vi "Test_UserEvent.vi"() -> (2 "Tests":cluster{"Test":string, "Passed":bool}[](array[cluster]), 3 "All Passed":bool)   [LabVIEW 2021]
uses:
  e99ad325-cf06-43e8-8912-3f55b24ea7fa.vi
  a4f08420-5a93-4bb2-8b8a-0d8211cb65b1.vi
  ced33e94-6682-457b-8286-a1586b91d3ac.vi
  d51e5e44-ed24-4473-837c-d660af8d3c6c.vi
  83069767-f90e-45e3-a161-ecb419ffe951.vi
  f3f8c4a7-11c8-469f-8d5b-86617bd7b3fe.vi
  09deaf97-c7a2-464e-bc40-56413b5f2ca1.vi
  a52824a8-f54c-45d4-a385-e62717a03234.vi
  a41de4ac-8db4-49b3-973c-25645465983a.vi
  f14a211d-4f31-4d7c-a2ff-2b54c0eab8a5.vi
  ee9b06b6-63a8-446a-8c72-f25155a75d2f.vi
  463acd0f-6dc2-4dbc-9232-112ef0c236db.vi
  653d2893-4bda-4f3e-a7e2-69abc9b10a93.vi
  759f70c8-bf56-4c58-9cd1-cbf254d2a4d5.vi
  cc1a389b-89ef-4407-98bb-40b68853af6d.vi
  74880120-8c1e-4130-96c5-fbcdd9dfdcb0.vi
  1ce71085-c310-4f8b-ab8a-af74af3ddc51.vi
  src/SubVIs/Map.vi
  <vilib>/Utility/error.llb/Error Cluster From Error Code.vi
  <vilib>/ErrorRing/Error Ring.xnode
  src/UserEvent.lvlib
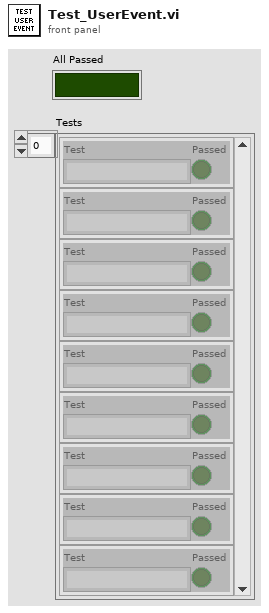
[diagram p1: front panel]
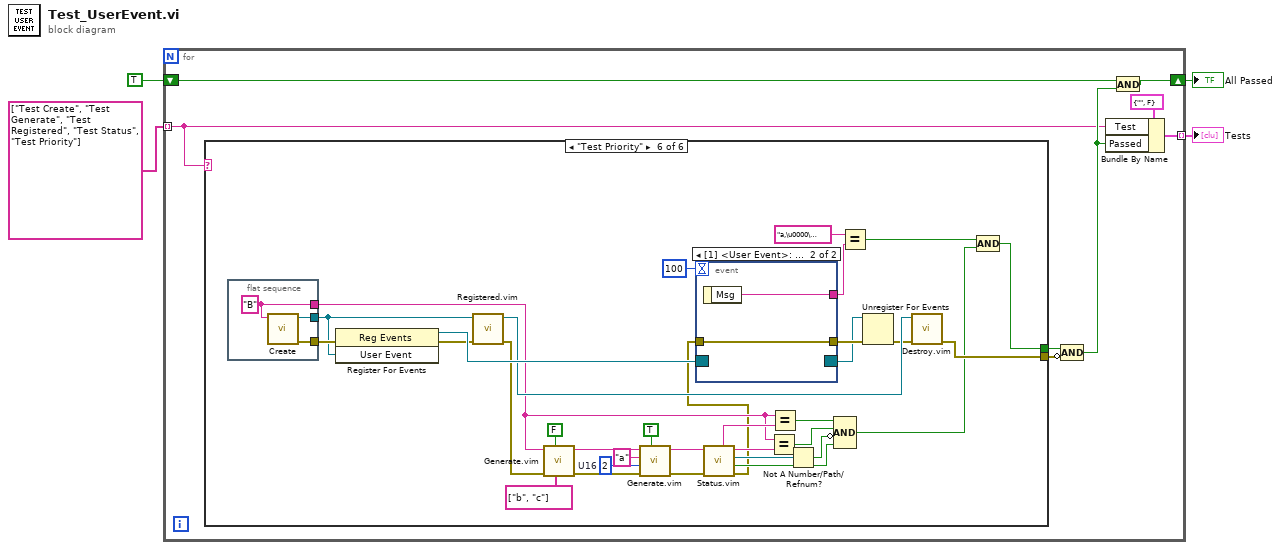
[diagram p0: block diagram]
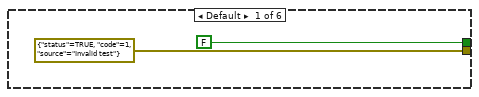
[diagram p2: hidden frame]
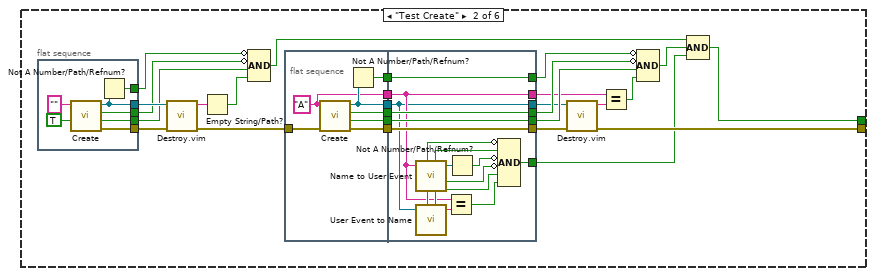
[diagram p3: hidden frame]
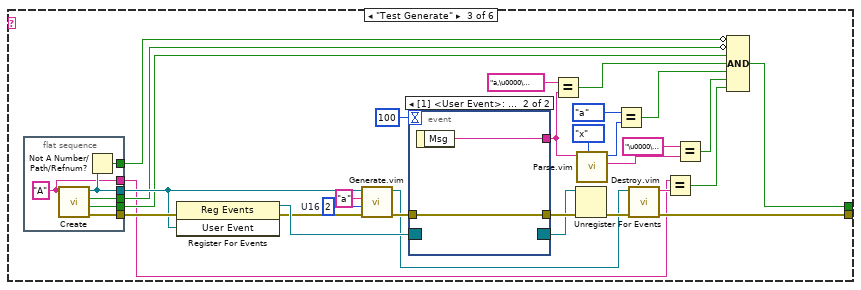
[diagram p4: hidden frame]
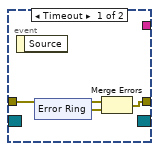
[diagram p5: hidden frame]
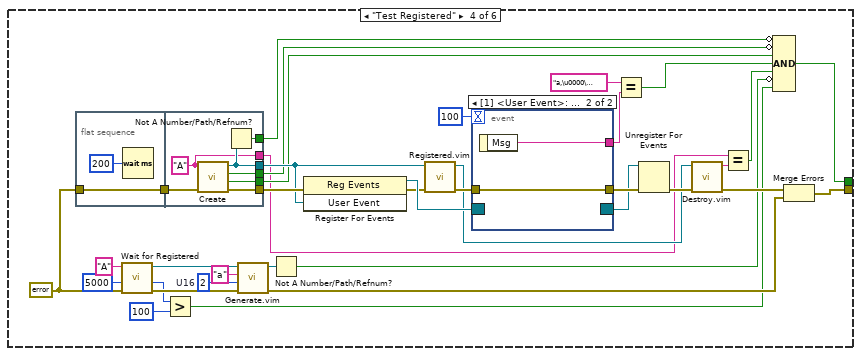
[diagram p6: hidden frame]
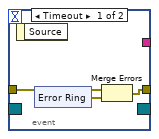
[diagram p7: hidden frame]
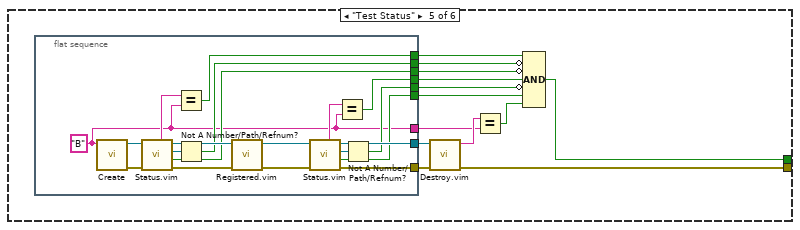
[diagram p8: hidden frame]
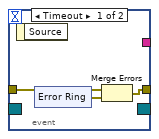
[diagram p9: hidden frame]
diagram:
  n1 = for {
    shift-right: [w11] -> w1
    shift-left: TRUE -> [w12]
    tunnel: string[] ["Test Create", "Test Generate", "Test Registered", "Test Status", "Test Priority"] -> [w6] mode=indexing
    tunnel: [w7] -> w2 mode=indexing
    n2 = case shown="\"Test Priority\"" w6 {
      tunnel: [errorcluster {"status"=TRUE, "code"=1, "source"="Invalid test"} ("error in (no error)") w23 w99 w120 w180 w210] -> w10
      tunnel: [FALSE w22 w79 w131 w170 w208] -> w5
      frame Default {
      }
      frame "Test Create" {
        n3 = flat-sequence {
          tunnel: [w68] -> w41
          tunnel: [w67] -> w40
          tunnel: [w66] -> w38
          tunnel: [w65] -> w37
          tunnel: [w64] -> w36
          frame #0 {
            n4 = call "Create.vi"("Create if not Found? (T)"=TRUE, "User Event Name (\"\"=Unnamed)"="" ("User Event Name (\"\"=Unnamed)")) -> ("error out"=w68:errorcluster, "Created New?"=w64:bool, "Is Registered?"=w65:bool, "User Event"=w67:refnum<user-event>)  [unwired: 6 in]
            n5 = Not A Number/Path/Refnum?(number/path/refnum=w67) -> (NaN/Path/Refnum?=w66:bool)
          }
        }
        n6 = call "Destroy.vim"("error in (no error)"=w41, "User Event in"=w40) -> ("error out"=w29:errorcluster, "User Event Name"=w39:string)  [unwired: 8 in]
        n7 = Empty String/Path?(string/path=w39) -> (empty?=w35:bool)
        n8 = Compound Arithmetic op=AND(invert w38, invert w37, w36, w35) -> (w24:bool)
        n9 = flat-sequence {
          tunnel: w29 -> [w44]
          tunnel: [w48] -> w20
          tunnel: [w47] -> w19
          tunnel: [w46] -> w18
          tunnel: [w43] -> w17
          tunnel: [w45] -> w16
          tunnel: [w42] -> w15
          tunnel: [w51] -> w21
          tunnel: [w50] -> w27
          tunnel: [w60] -> w30
          tunnel: [w49] -> w31
          tunnel: [w61] -> w32
          tunnel: [w62] -> w33
          tunnel: [w63] -> w34
          tunnel: w20 -> [w63]
          tunnel: w19 -> [w62]
          tunnel: w18 -> [w61]
          tunnel: w17 -> [w49]
          tunnel: w16 -> [w60]
          tunnel: w15 -> [w50]
          frame #0 {
            w42 = "A" ("User Event Name (\"\"=Unnamed)")
            n10 = call "Create.vi"("error in (no error)"=w44, "User Event Name (\"\"=Unnamed)"=w42) -> ("error out"=w45:errorcluster, "Created New?"=w48:bool, "Is Registered?"=w47:bool, "User Event"=w43:refnum<user-event>)  [unwired: 6 in]
            n11 = Not A Number/Path/Refnum?(number/path/refnum=w43) -> (NaN/Path/Refnum?=w46:bool)
          }
          frame #1 {
            n12 = call "Name to User Event.vi"("User Event Name"=w50) -> ("Is Registered?"=w52:bool, "Found?"=w53:bool, "User Event"=w54:refnum<user-event>)  [unwired: 6 in]
            n13 = call "User Event to Name.vi"("User Event"=w49) -> ("Is Registered?"=w57:bool, "Found?"=w58:bool, "User Event Name"=w56:string)  [unwired: 6 in]
            n14 = Equal?(x=w50, y=w56) -> (x = y?=w59:bool)
            n15 = Not A Number/Path/Refnum?(number/path/refnum=w54) -> (NaN/Path/Refnum?=w55:bool)
            n16 = Compound Arithmetic op=AND(invert w52, w53, invert w55, invert w57, w58, w59) -> (w51:bool)
          }
        }
        n17 = call "Destroy.vim"("error in (no error)"=w30, "User Event in"=w31) -> ("error out"=w23:errorcluster, "User Event Name"=w28:string)  [unwired: 8 in]
        n18 = Equal?(x=w27, y=w28) -> (x = y?=w26:bool)
        n19 = Compound Arithmetic op=AND(invert w32, invert w33, w34, w26) -> (w25:bool)
        n20 = Compound Arithmetic op=AND(w24, w25, w21) -> (w22:bool)
      }
      frame "Test Generate" {
        w89 = u16 2  # U16
        n21 = flat-sequence {
          tunnel: [w115] -> w84
          tunnel: [w114] -> w85
          tunnel: [w113] -> w86
          tunnel: [w112] -> w90
          tunnel: [w111] -> w100
          tunnel: [w110] -> w81
          frame #0 {
            w110 = "A" ("User Event Name (\"\"=Unnamed)")
            n22 = call "Create.vi"("User Event Name (\"\"=Unnamed)"=w110) -> ("error out"=w111:errorcluster, "Created New?"=w115:bool, "Is Registered?"=w114:bool, "User Event"=w112:refnum<user-event>)  [unwired: 7 in]
            n23 = Not A Number/Path/Refnum?(number/path/refnum=w112) -> (NaN/Path/Refnum?=w113:bool)
          }
        }
        n24 = register-events(error in=w100, w90) -> (reference out=w97:refnum<event-registration>, error out=w93:errorcluster)  [unwired: 1 in]
        n25 = call "Generate.vim"("error in (no error)"=w93, "Data"=w89, "Message"="a", "User Event in"=w90) -> ("error out"=w92:errorcluster, "User Event"=w88:refnum<user-event>)  [unwired: 6 in]
        n26 = event shown="[1] <User Event>: User Event" {
          selector: w97 -> [_ _]
          dyn-events: [_ _] -> w95
          timeout: 100 -> [_ _]
          tunnel: [w102 w109] -> w98
          tunnel: w92 -> [w103 w109]
          tunnel: [_ w108] -> w77
          event Timeout {
            n27 = event-data() -> ()  [unwired: 1 in, 1 out]
            n28 = xnode "Error Ring"() -> ("error out"=w101:errorcluster)
            n29 = Merge Errors(w103, w101) -> (w102:errorcluster)
          }
          event User Event {
            n30 = event-data() -> ("Msg"=w108:string)  [unwired: 1 in]
          }
        }
        n31 = Equal?(x="a,\u0000\u0002", y=w77) -> (x = y?=w83:bool)
        n32 = Unregister For Events(event registration refnum=w95, error in=w98) -> (error out=w96:errorcluster)
        n33 = call "Parse.vim"("Message Type"=enum16{"x", "a", "b"}."x", "Msg"=w77) -> ("Data out"=w74:string, "Message out"=w75:enum16{"x", "a", "b"})  [unwired: 8 in]
        n34 = Equal?(x=enum16{"x", "a", "b"}."a", y=w75) -> (x = y?=w72:bool)
        n35 = call "Destroy.vim"("error in (no error)"=w96, "User Event in"=w88) -> ("error out"=w99:errorcluster, "User Event Name"=w82:string)  [unwired: 8 in]
        n36 = Equal?(x=w81, y=w82) -> (x = y?=w80:bool)
        n37 = Equal?(x="\u0000\u0002", y=w74) -> (x = y?=w71:bool)
        n38 = Compound Arithmetic op=AND(invert w86, invert w85, w84, w83, w72, w71, w80) -> (w79:bool)
      }
      frame "Test Registered" {
        w121 = u16 2  # U16
        w128 = errorcluster {"status"=FALSE, "code"=0, "source"=""} ("error in (no error)")
        n39 = flat-sequence {
          tunnel: [w161] -> w129
          tunnel: w128 -> [w161]
          tunnel: [w169] -> w136
          tunnel: [w168] -> w137
          tunnel: [w167] -> w138
          tunnel: [w166] -> w142
          tunnel: [w165] -> w151
          tunnel: [w164] -> w133
          tunnel: w129 -> [w163]
          frame #0 {
            n40 = Wait (ms)(milliseconds to wait=u32 200) -> ()  [unwired: 1 out]
          }
          frame #1 {
            w164 = "A" ("User Event Name (\"\"=Unnamed)")
            n41 = call "Create.vi"("error in (no error)"=w163, "User Event Name (\"\"=Unnamed)"=w164) -> ("error out"=w165:errorcluster, "Created New?"=w169:bool, "Is Registered?"=w168:bool, "User Event"=w166:refnum<user-event>)  [unwired: 6 in]
            n42 = Not A Number/Path/Refnum?(number/path/refnum=w166) -> (NaN/Path/Refnum?=w167:bool)
          }
        }
        n43 = call "Wait for Registered.vi"("error in (no error)"=w128, "ms Timeout (5000)"=u32 5000, "User Event Name"="A") -> ("error out"=w130:errorcluster, "ms Elapsed"=w124:u32, "User Event"=w125:refnum<user-event>)  [unwired: 6 in]
        n44 = Greater?(x=w124, y=u32 100) -> (0:w116:bool)
        n45 = call "Generate.vim"("error in (no error)"=w130, "Data"=w121, "Message"="a", "User Event in"=w125) -> ("error out"=w119:errorcluster, "User Event"=w118:refnum<user-event>)  [unwired: 6 in]
        n46 = Not A Number/Path/Refnum?(number/path/refnum=w118) -> (NaN/Path/Refnum?=w117:bool)
        n47 = register-events(error in=w151, w142) -> (reference out=w148:refnum<event-registration>, error out=w144:errorcluster)  [unwired: 1 in]
        n48 = call "Registered.vim"("error in (no error)"=w144, "User Event in"=w142) -> ("error out"=w143:errorcluster, "User Event"=w141:refnum<user-event>)  [unwired: 8 in]
        n49 = event shown="[1] <User Event>: User Event" {
          selector: w148 -> [_ _]
          dyn-events: [_ _] -> w146
          timeout: 100 -> [_ _]
          tunnel: [w153 w159] -> w149
          tunnel: w143 -> [w154 w159]
          tunnel: [_ w160] -> w140
          event Timeout {
            n50 = event-data() -> ()  [unwired: 1 in, 1 out]
            n51 = xnode "Error Ring"() -> ("error out"=w152:errorcluster)
            n52 = Merge Errors(w154, w152) -> (w153:errorcluster)
          }
          event User Event {
            n53 = event-data() -> ("Msg"=w160:string)  [unwired: 1 in]
          }
        }
        n54 = Equal?(x="a,\u0000\u0002", y=w140) -> (x = y?=w135:bool)
        n55 = Unregister For Events(event registration refnum=w146, error in=w149) -> (error out=w147:errorcluster)
        n56 = call "Destroy.vim"("error in (no error)"=w147, "User Event in"=w141) -> ("error out"=w150:errorcluster, "User Event Name"=w134:string)  [unwired: 8 in]
        n57 = Equal?(x=w133, y=w134) -> (x = y?=w132:bool)
        n58 = Compound Arithmetic op=AND(invert w138, invert w137, w136, w135, w132, invert w117, w116) -> (w131:bool)
        n59 = Merge Errors(w150, w119) -> (w120:errorcluster)
      }
      frame "Test Status" {
        n60 = flat-sequence {
          tunnel: [w195] -> w182
          tunnel: [w194] -> w181
          tunnel: [w193] -> w179
          tunnel: [w191] -> w178
          tunnel: [w189] -> w177
          tunnel: [w187] -> w176
          tunnel: [w185] -> w175
          tunnel: [w184] -> w174
          tunnel: [w183] -> w172
          frame #0 {
            w183 = "B" ("User Event Name (\"\"=Unnamed)")
            n61 = call "Create.vi"("User Event Name (\"\"=Unnamed)"=w183) -> ("error out"=w201:errorcluster, "User Event"=w200:refnum<user-event>)  [unwired: 7 in, 2 out]
            n62 = call "Status.vim"("error in (no error)"=w201, "User Event in"=w200) -> ("error out"=w198:errorcluster, "Is Registered?"=w193:bool, "User Event"=w192:refnum<user-event>, "User Event out"=w199:refnum<user-event>, "User Event Name"=w190:string)  [unwired: 5 in]
            n63 = Equal?(x=w190, y=w183) -> (x = y?=w189:bool)
            n64 = Not A Number/Path/Refnum?(number/path/refnum=w192) -> (NaN/Path/Refnum?=w191:bool)
            n65 = call "Registered.vim"("error in (no error)"=w198, "User Event in"=w199) -> ("error out"=w196:errorcluster, "User Event"=w197:refnum<user-event>)  [unwired: 8 in]
            n66 = call "Status.vim"("error in (no error)"=w196, "User Event in"=w197) -> ("error out"=w195:errorcluster, "Is Registered?"=w184:bool, "User Event"=w186:refnum<user-event>, "User Event out"=w194:refnum<user-event>, "User Event Name"=w188:string)  [unwired: 5 in]
            n67 = Equal?(x=w188, y=w183) -> (x = y?=w187:bool)
            n68 = Not A Number/Path/Refnum?(number/path/refnum=w186) -> (NaN/Path/Refnum?=w185:bool)
          }
        }
        n69 = call "Destroy.vim"("error in (no error)"=w182, "User Event in"=w181) -> ("error out"=w180:errorcluster, "User Event Name"=w173:string)  [unwired: 8 in]
        n70 = Equal?(x=w173, y=w172) -> (x = y?=w171:bool)
        n71 = Compound Arithmetic op=AND(w177, invert w178, invert w179, w176, invert w175, w174, w171) -> (w170:bool)
      }
      frame "Test Priority" {
        w226 = u16 2  # U16
        n72 = flat-sequence {
          tunnel: [w247] -> w229
          tunnel: [w246] -> w228
          tunnel: [w245] -> w206
          frame #0 {
            w245 = "B" ("User Event Name (\"\"=Unnamed)")
            n73 = call "Create.vi"("User Event Name (\"\"=Unnamed)"=w245) -> ("error out"=w247:errorcluster, "User Event"=w246:refnum<user-event>)  [unwired: 7 in, 2 out]
          }
        }
        n74 = register-events(error in=w229, w228) -> (reference out=w234:refnum<event-registration>, error out=w219:errorcluster)  [unwired: 1 in]
        n75 = call "Registered.vim"("error in (no error)"=w219, "User Event in"=w228) -> ("error out"=w203:errorcluster, "User Event"=w231:refnum<user-event>)  [unwired: 8 in]
        n76 = call "Generate.vim"("Messages"=string[] ["b", "c"], "Priority? (F)"=FALSE, "error in (no error)"=w203, "User Event in"=w206) -> ("error out"=w220:errorcluster, "User Event"=w218:string)  [unwired: 6 in]
        n77 = call "Generate.vim"("Priority? (F)"=TRUE, "error in (no error)"=w220, "Data"=w226, "Message"="a", "User Event in"=w218) -> ("error out"=w224:errorcluster, "User Event"=w223:string)  [unwired: 5 in]
        n78 = call "Status.vim"("error in (no error)"=w224, "User Event in"=w223) -> ("error out"=w202:errorcluster, "Is Registered?"=w211:bool, "User Event"=w214:refnum<user-event>, "User Event out"=w207:string, "User Event Name"=w215:string)  [unwired: 5 in]
        n79 = event shown="[1] <User Event>: User Event" {
          selector: w234 -> [_ _]
          dyn-events: [_ _] -> w233
          timeout: 100 -> [_ _]
          tunnel: [w237 w243] -> w235
          tunnel: w202 -> [w238 w243]
          tunnel: [_ w244] -> w225
          event Timeout {
            n80 = event-data() -> ()  [unwired: 1 in, 1 out]
            n81 = xnode "Error Ring"() -> ("error out"=w236:errorcluster)
            n82 = Merge Errors(w238, w236) -> (w237:errorcluster)
          }
          event User Event {
            n83 = event-data() -> ("Msg"=w244:string)  [unwired: 1 in]
          }
        }
        n84 = Equal?(x=w206, y=w207) -> (x = y?=w205:bool)
        n85 = Equal?(x=w206, y=w215) -> (x = y?=w213:bool)
        n86 = Not A Number/Path/Refnum?(number/path/refnum=w214) -> (NaN/Path/Refnum?=w212:bool)
        n87 = Compound Arithmetic op=AND(w213, w205, invert w212, w211) -> (w209:bool)
        n88 = Equal?(x="a,\u0000\u0002", y=w225) -> (x = y?=w216:bool)
        n89 = Unregister For Events(event registration refnum=w233, error in=w235) -> (error out=w204:errorcluster)
        n90 = call "Destroy.vim"("error in (no error)"=w204, "User Event in"=w231) -> ("error out"=w210:errorcluster)  [unwired: 8 in, 1 out]
        n91 = Compound Arithmetic op=AND(w216, w209) -> (w208:bool)
      }
    }
    n92 = Compound Arithmetic op=AND(w5, invert w10) -> (w8:bool)
    n93 = Bundle By Name(cluster=cluster{"Test":string, "Passed":bool} {"Test"="", "Passed"=FALSE} ("Cluster"), "Test"=w6, "Passed"=w8) -> (w7:cluster{"Test":string, "Passed":bool})
    n94 = And(x=w12, y=w8) -> (x .and. y?=w11:bool)
  }
  "All Passed" <- w1
  "Tests" <- w2
